vi "delta initalize read(SubVI).vi"(9 "字符串":string, 11 "队列输出":refnum<queue>) -> (1 "2812 -A Params Out":T6={"Auto Range?"=FALSE, "Man / Selected\nRange"=enum."10mV", "Enable Digital\nFilter?"=FALSE, "Filter Type"=enum."Moving", "Filter Count"=10, "Filter\nWindow (%)"=0.01, "Enable Analog\nFilter?"=FALSE, "NPLCs"=5} {"Filter\nWindow (%)" min=0.0 max=10.0 step=0.01 format="%.2f"; "Filter Count" min=1 max=100; "NPLCs" min=1 max=10}, 2 "Delta Mode Params Out":T7={"High Level (A)"=0.001, "Low Level (A)"=-0.001, "Delay (s)"=0.002, "Num Cycles Mode"=enum."Finite Count", "Finite Count"=1, "Abort On\nCompliance?"=FALSE, "Cold Swithing\nMode Enabled?"=FALSE} {"Finite Count" min=1 max=65536; "Low Level (A)" min=-0.105 max=0.0 format="%.3p"; "High Level (A)" min=0.0 max=0.105 format="%.3p"; "Delay (s)" min=0.001 max=9999.999 format="%.3f"}, 3 "6221 Resource Out":refnum<visa-resource-name>="GPIB0::24::INSTR")   [LabVIEW 2019, in "SubVI.lvlib"]
uses:
  SubVI.lvlib
  lib/Keithley 622x/Configure/Delta PDelta DCon Modes/Typedefs/KE622x -- Delta Mode Params.ctl
  lib/Keithley 622x/Configure/Delta PDelta DCon Modes/Low Level/Typedefs/KE622x -- Delta PDelta Mode High Level.ctl
  lib/Keithley 622x/Configure/Delta PDelta DCon Modes/Low Level/Typedefs/KE622x -- Delta PDelta Mode Low Level.ctl
  lib/Keithley 622x/Configure/Delta PDelta DCon Modes/Low Level/Typedefs/KE622x -- Delta DCon Mode Delay.ctl
  lib/Keithley 622x/Configure/Delta PDelta DCon Modes/Low Level/Typedefs/KE622x -- Delta PDelta Mode Num Cycles Mode.ctl
  lib/Keithley 622x/Configure/Delta PDelta DCon Modes/Low Level/Typedefs/KE622x -- Delta PDelta Mode Num Cycles.ctl
  lib/Keithley 622x/Configure/2182 -A/Low Level/Typedefs/KE2182 -- Voltage Ranges.ctl
  lib/Keithley 622x/Configure/2182 -A/Low Level/Typedefs/KE2182 -- Filter Type.ctl
  lib/Keithley 622x/Configure/2182 -A/Low Level/Typedefs/KE2182 -- Filter Count.ctl
  lib/Keithley 622x/Configure/2182 -A/Low Level/Typedefs/KE2182 -- Filter Window.ctl
  lib/Keithley 622x/Configure/2182 -A/Low Level/Typedefs/KE2182 -- NPLCs.ctl
  config.ctl
  lib/Keithley 622x/Keithley 622x.lvlib
panel:
  in  "2812 -A Params In":T6={"Auto Range?"=FALSE, "Man / Selected\nRange"=enum."10mV", "Enable Digital\nFilter?"=FALSE, "Filter Type"=enum."Moving", "Filter Count"=10, "Filter\nWindow (%)"=0.01, "Enable Analog\nFilter?"=FALSE, "NPLCs"=5} {"Filter\nWindow (%)" min=0.0 max=10.0 step=0.01 format="%.2f"; "Filter Count" min=1 max=100; "NPLCs" min=1 max=10}
  in  "Delta Mode Params In":T7={"High Level (A)"=0.001, "Low Level (A)"=-0.001, "Delay (s)"=0.002, "Num Cycles Mode"=enum."Finite Count", "Finite Count"=1, "Abort On\nCompliance?"=FALSE, "Cold Swithing\nMode Enabled?"=FALSE} {"Finite Count" min=1 max=65536; "Low Level (A)" min=-0.105 max=0.0 format="%.3p"; "High Level (A)" min=0.0 max=0.105 format="%.3p"; "Delay (s)" min=0.001 max=9999.999 format="%.3f"}
  in  "6221 Resource":refnum<visa-resource-name>="GPIB0::24::INSTR"
  # "(真是通道1，假是通道2)"
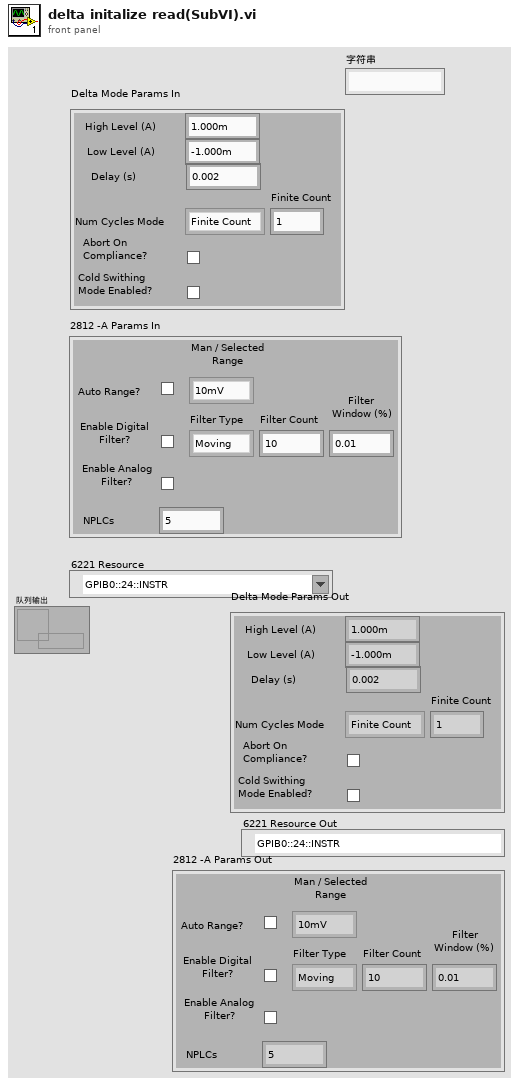
[diagram p1: front panel]
types:
  T1 = typedef "Keithley 622x.lvlib/KE2182 -- Voltage Ranges.ctl" = enum16{"10mV", "100mV", "1V", "10V", "100V"}
  T2 = typedef "Keithley 622x.lvlib/KE2182 -- Filter Type.ctl" = enum16{"Moving", "Repeat"}
  T3 = typedef "Keithley 622x.lvlib/KE2182 -- Filter Count.ctl" = u32
  T4 = typedef "Keithley 622x.lvlib/KE2182 -- Filter Window.ctl" = dbl
  T5 = typedef "Keithley 622x.lvlib/KE2182 -- NPLCs.ctl" = u32
  T6 = cluster{"Auto Range?":bool, "Man / Selected\nRange":T1, "Enable Digital\nFilter?":bool, "Filter Type":T2, "Filter Count":T3, "Filter\nWindow (%)":T4, "Enable Analog\nFilter?":bool, "NPLCs":T5}
  T7 = typedef "Keithley 622x.lvlib/KE622x -- Delta Mode Params.ctl" = cluster{"High Level (A)":T8, "Low Level (A)":T9, "Delay (s)":T10, "Num Cycles Mode":T11, "Finite Count":T12, "Abort On\nCompliance?":bool, "Cold Swithing\nMode Enabled?":bool}
  T8 = typedef "Keithley 622x.lvlib/KE622x -- Delta PDelta Mode High Level.ctl" = dbl
  T9 = typedef "Keithley 622x.lvlib/KE622x -- Delta PDelta Mode Low Level.ctl" = dbl
  T10 = typedef "Keithley 622x.lvlib/KE622x -- Delta DCon Mode Delay.ctl" = dbl
  T11 = typedef "Keithley 622x.lvlib/KE622x -- Delta PDelta Mode Num Cycles Mode.ctl" = enum16{"Finite Count", "Infinite"}
  T12 = typedef "Keithley 622x.lvlib/KE622x -- Delta PDelta Mode Num Cycles.ctl" = u32
  T13 = enum16{"open", "replace", "create", "open or create", "replace or create", "replace or create with confirmation"}
  T14 = typedef "config.ctl" = cluster{"error":bool, "initialize":string, "数值":dbl, "6221":cluster{"6221 Resource":refnum<visa-resource-name>, "Delta status":bool}, "7001":cluster{"Ch":bool}}
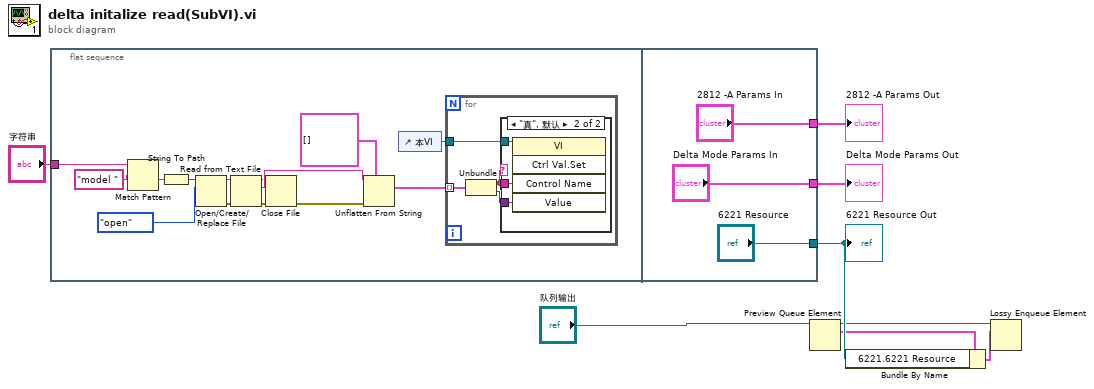
[diagram p0: block diagram]
diagram:
  n1 = flat-sequence {
    tunnel: "字符串" -> [w22]
    tunnel: ["Delta Mode Params In"] -> w7
    tunnel: ["6221 Resource"] -> w4
    tunnel: ["2812 -A Params In"] -> w6
    frame #0 {
      n2 = Match Pattern(string=w22, regular expression="model " ("正则表达式")) -> (after substring=w21:string)  [unwired: 1 in, 3 out]
      n3 = String To Path(string=w21) -> (path=w20:path)
      n4 = Open/Create/Replace File(file path (use dialog)=w20, operation (0:open)=T13."open" ("操作(0:open)")) -> (refnum out=w17:refnum<file>, error out=w15:errorcluster)  [unwired: 4 in, 1 out]
      n5 = Read from Text File(file (use dialog)=w17, error in=w15) -> (refnum out=w16:refnum<file>, text=w18:string, error out=w14:errorcluster)  [unwired: 2 in, 1 out]
      n6 = Close File(refnum=w16, error in=w14) -> (error out=w13:errorcluster)  [unwired: 1 out]
      n7 = Unflatten From String(type=cluster{"Name":string, "Variant Data":variant}[] [] ("控件值:获取全部"), binary string=w18, error in (no error)=w13) -> (value=w10:cluster{"Name":string, "Variant Data":variant}[])  [unwired: 2 in, 2 out]
      n8 = control-ref of="本VI"() -> (w9:refnum<vi>)
      n9 = for {
        tunnel: w10 -> [w26] mode=indexing
        tunnel: w9 -> [w25]
        n10 = Unbundle(w26) -> ("Name"=w23:string, "Variant Data"=w24:variant)
        n11 = case shown="\"真\", 默认" w23 {
          tunnel: w25 -> [_ w29]
          tunnel: w23 -> [_ w28]
          tunnel: w24 -> [_ w27]
          frame "cancel", "load", "ok" {
          }
          frame "真", Default {
            n12 = invoke class="VI" method="Ctrl Val.Set"(reference=w29, "Control Name"=w28, "Value"=w27) -> ()  [unwired: 2 in, 5 out]
          }
        }
      }
    }
    frame #1 {
    }
  }
  n13 = Preview Queue Element(queue="队列输出") -> (queue out=w2:refnum<queue>, element=w3:T14)  [unwired: 2 in, 2 out]
  n14 = Bundle By Name(cluster=w3, "6221.6221 Resource"=w4) -> (w1:T14)
  n15 = Lossy Enqueue Element(queue=w2, element=w1) -> ()  [unwired: 1 in, 4 out]
  "Delta Mode Params Out" <- w7
  "6221 Resource Out" <- w4
  "2812 -A Params Out" <- w6
